vi "Send CCD Status.vi"(8 "error in (no error)":errorcluster, 11 "RxTx in":refnum<class "RxTx.lvclass">) -> (0 "error out":errorcluster, 3 "RxTx out":refnum<class "RxTx.lvclass">)   [LabVIEW 2018, in "RxTx.lvclass"]
uses:
  RxTx.lvclass
  RxTx.lvclass/RxTx.ctl
  Interface/Interface.lvclass
  <vilib>/Utility/Data Type/NI_Data Type.lvlib
panel:
  out "Camera Status 2":T1
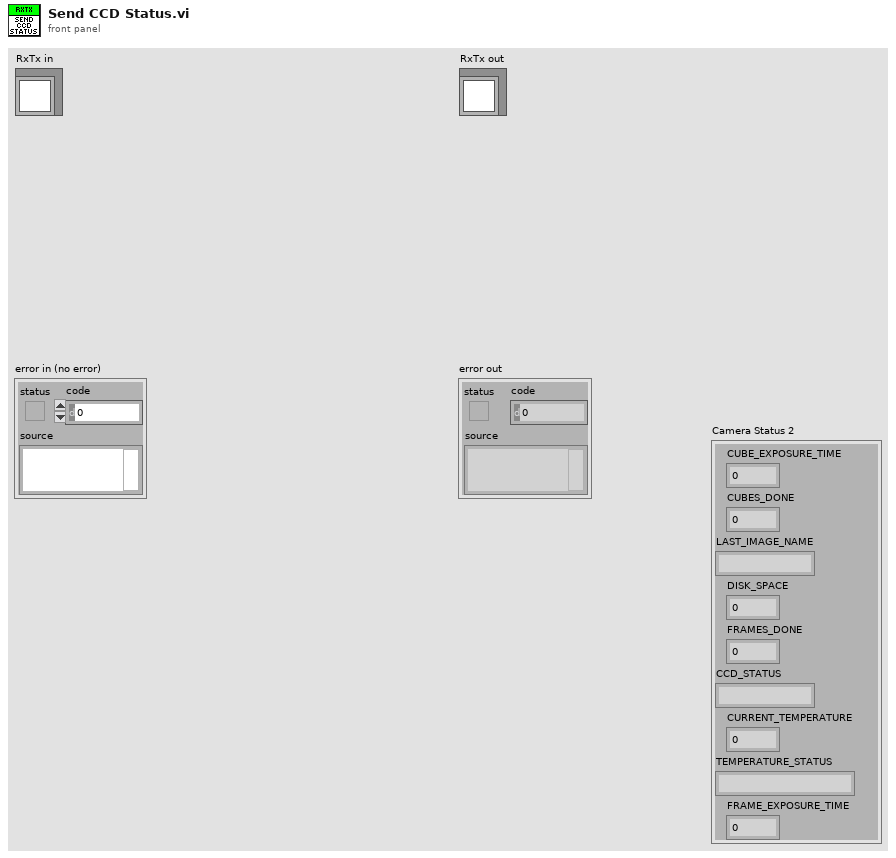
[diagram p1: front panel]
types:
  T1 = cluster{"CUBE_EXPOSURE_TIME":sgl, "CUBES_DONE":u16, "LAST_IMAGE_NAME":string, "DISK_SPACE":u16, "FRAMES_DONE":u16, "CCD_STATUS":string, "CURRENT_TEMPERATURE":i16, "TEMPERATURE_STATUS":string, "FRAME_EXPOSURE_TIME":u16}
  T2 = cluster{"CUBE_EXPOSURE_TIME":sgl, "CUBES_DONE":u16, "LAST_IMAGE_NAME":string, "DISK_SPACE":u16, "FRAMES_DONE":u16, "CCD_STATUS":string, "CURRENT_TEMPERATURE":i16, "TEMPERATURE_STATUS":string, "FRAME_EXPOSURE_TIME":u16, "CCD_ON_OFF":bool, "SERIAL_NUMBER":u16, "ACQUIRING":bool}
  T3 = typedef "NI_Data Type.lvlib/Data Type.ctl" = enum8{"Invalid Type", "Void", "I8", "I16", "I32", "I64", "U8", "U16", "U32", "U64", "Single Float", "Double Float", "Extended Float", "Single Complex", "Double Complex", "Extended Complex", "Enum U8", "Enum U16", "Enum U32", "Enum U64", "Single Float With Unit", "Double Float With Unit", "Extended Float With Unit", "Single Complex with Unit", "Double Complex with Unit", "Extended Complex with Unit", "Boolean", "String", "Path", "Picture", "Tag", "Array", "Cluster", "Variant", "LV Variant", "Waveform", "Timestamp", "Digital Waveform", "Digital Data", "ExpressData", "Refnum", "External Data", "VI", "Poly VI", "LabVIEW Class Instance", "Fixed Point"}
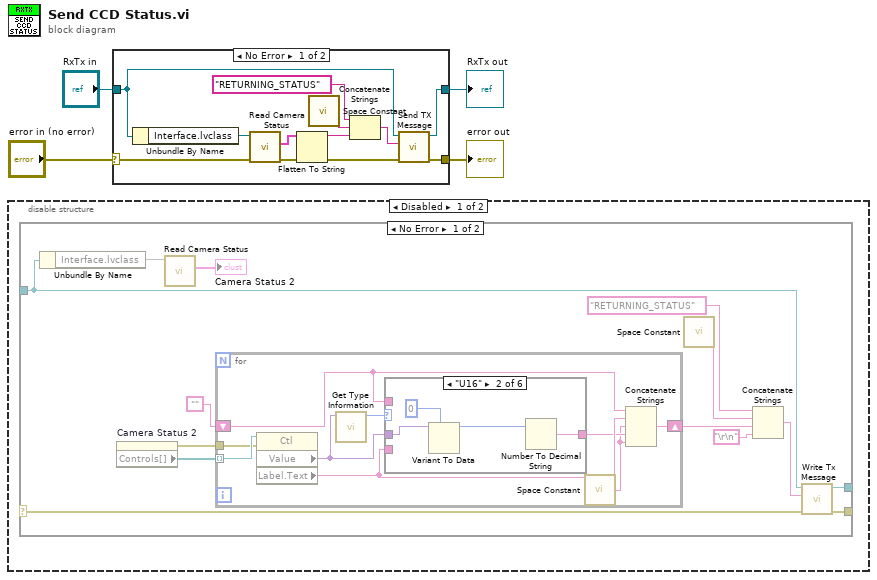
[diagram p0: block diagram]
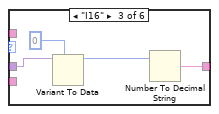
[diagram p3: hidden frame]
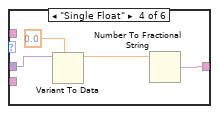
[diagram p4: hidden frame]
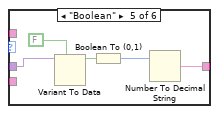
[diagram p5: hidden frame]
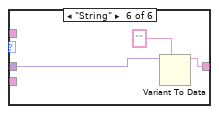
[diagram p6: hidden frame]
diagram:
  n1 = disable-structure shown="Disabled" {
    frame Disabled {
      n2 = case shown="No Error" {
        selector: _ -> [w17 w49]
        tunnel: [w12 w49] -> _
        tunnel: [w13 w48] -> _
        tunnel: _ -> [w14 w48]
        frame No Error {
          n3 = Unbundle By Name(w14) -> ("Interface.lvclass"=w18)
          n4 = property on="Camera Status 2" class="Clust (strict)"() -> (error out=w6:errorcluster, "Controls[]"=w7:refnum<vi>[])  [unwired: 2 in, 1 out]
          n5 = call "Read Camera Status.vi"("Interface in"=w18) -> ("Camera Status"=→"Camera Status 2":T2)  [unwired: 8 in, 2 out]
          n6 = for {
            shift-right: [w22] -> w16
            shift-left: "" -> [w24]
            tunnel: w7 -> [w20] mode=indexing
            tunnel: w6 -> [w19]
            n7 = property class="Ctl"(reference=w20, error in=w19) -> ("Value"=w26:variant, "Label.Text"=w25:string)  [unwired: 2 out]
            n8 = call <vilib>:"Get Type Information.vi"("Variant"=w26) -> ("Type"=w27:T3)  [unwired: 6 in, 4 out]
            n9 = case shown="\"U16\"" w27 {
              tunnel: w26 -> [_ w31 w35 w39 w44 w46]
              tunnel: w25 -> [_ _ _ _ _ _]
              tunnel: w24 -> [_ _ _ _ _ _]
              tunnel: [_ w28 w32 w36 w40 w45] -> w23
              frame "Invalid Type", Default {
              }
              frame "U16" {
                n10 = Variant To Data(type=u16 0, Variant=w31) -> (data=w29:u16)  [unwired: 1 in, 1 out]
                n11 = Number To Decimal String(number=w29) -> (decimal integer string=w28:string)  [unwired: 1 in]
              }
              frame "I16" {
                n12 = Variant To Data(type=i16 0, Variant=w35) -> (data=w33:i16)  [unwired: 1 in, 1 out]
                n13 = Number To Decimal String(number=w33) -> (decimal integer string=w32:string)  [unwired: 1 in]
              }
              frame "Single Float" {
                n14 = Variant To Data(type=sgl 0.0, Variant=w39) -> (data=w37:sgl)  [unwired: 1 in, 1 out]
                n15 = Number To Fractional String(number=w37) -> (F-format string=w36:string)  [unwired: 3 in]
              }
              frame "Boolean" {
                n16 = Variant To Data(type=FALSE, Variant=w44) -> (data=w42:bool)  [unwired: 1 in, 1 out]
                n17 = Boolean To (0,1)(Boolean=w42) -> (0, 1=w41:i16)
                n18 = Number To Decimal String(number=w41) -> (decimal integer string=w40:string)  [unwired: 1 in]
              }
              frame "String" {
                n19 = Variant To Data(type="", Variant=w46) -> (data=w45:string)  [unwired: 1 in, 1 out]
              }
            }
            n20 = call <vilib>:"Space Constant.vi"() -> ("String"=w21:string)
            n21 = Concatenate Strings(w24, w25, w21, w23, w21) -> (w22:string)
          }
          n22 = call <vilib>:"Space Constant.vi"() -> ("String"=w10:string)
          n23 = Concatenate Strings("RETURNING_STATUS", w10, w16, "\r\n") -> (w15:string)
          n24 = call "Write Tx Message.vi"("error in (no error)"=w17, "Tx Message"=w15, "RxTx in"=w14) -> ("error out"=w12:errorcluster, "RxTx out"=w13:refnum<class "RxTx.lvclass">)  [unwired: 7 in]
        }
        frame Error {
        }
      }
    }
    frame Enabled {
    }
  }
  n25 = case shown="No Error" "error in (no error)" {
    selector: "error in (no error)" -> [w55 w63]
    tunnel: [w50 w63] -> w2
    tunnel: [w51 w62] -> w1
    tunnel: "RxTx in" -> [w54 w62]
    frame No Error {
      n26 = Unbundle By Name(w54) -> ("Interface.lvclass"=w61:refnum<class "Interface.lvclass">)
      n27 = call "Read Camera Status.vi"("error in (no error)"=w55, "Interface in"=w61) -> ("error out"=w56:errorcluster, "Camera Status"=w58:T2)  [unwired: 7 in, 1 out]
      n28 = Flatten To String(anything=w58, error in (no error)=w56) -> (data string=w57:string, error out=w53:errorcluster)  [unwired: 2 in, 1 out]
      n29 = call <vilib>:"Space Constant.vi"() -> ("String"=w60:string)
      n30 = Concatenate Strings("RETURNING_STATUS", w60, w57) -> (w52:string)
      n31 = call "Send TX Message.vi"("error in (no error)"=w53, "element"=w52, "RxTx in"=w54) -> ("error out"=w50:errorcluster, "RxTx out"=w51:refnum<class "RxTx.lvclass">)  [unwired: 7 in]
    }
    frame Error {
    }
  }
  "error out" <- w2
  "RxTx out" <- w1
